vi "MCP4725 Example 1.vi"(8 "Error In":errorcluster) -> (0 "Error Out":errorcluster)   [LabVIEW 2014, in "LabVIEW Universal Transcriptor MCP4725.lvlib"]
uses:
  LabVIEW Universal Transcriptor MCP4725.lvlib
  MCP4725.lvclass
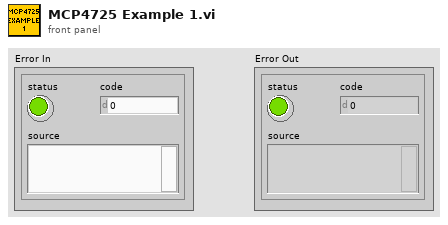
[diagram p1: front panel]
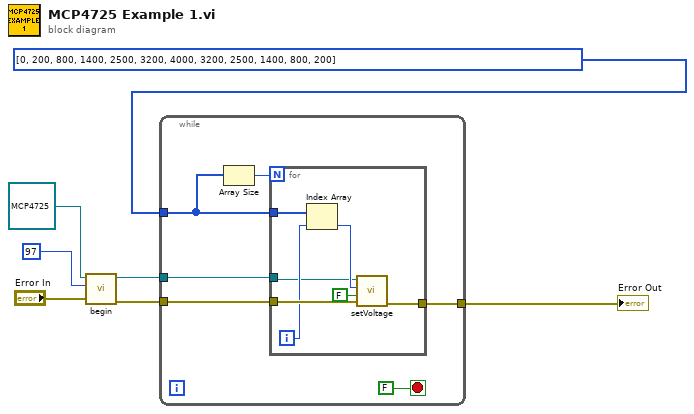
[diagram p0: block diagram]
diagram:
  n1 = call "begin.vi"("error in (no error)"="Error In", "I2C addr"=u8 97, "MCP4725 in"=refnum<class "MCP4725.lvclass"> refnum) -> ("error out"=w5:errorcluster, "MCP4725 out"=w4:refnum<class "MCP4725.lvclass">)  [unwired: 7 in]
  n2 = while {
    tunnel: w5 -> [w12]
    tunnel: w4 -> [w11]
    tunnel: u16[] [0, 200, 800, 1400, 2500, 3200, 4000, 3200, 2500, 1400, 800, 200] -> [w10]
    tunnel: [w8] -> w2
    stop <- FALSE stop-if-true
    n3 = Array Size(array=w10) -> (size(s)=w9:i32)
    n4 = for {
      N: w9 -> [_]
      tunnel: w12 -> [w20]
      tunnel: w11 -> [w16]
      tunnel: w10 -> [w19]
      tunnel: [w15] -> w8
      i -> [w18]
      n5 = Index Array(array=w19, index=w18) -> (element=w17:u16)
      n6 = call "setVoltage.vi"("error in (no error)"=w20, "writeEEPROM?"=FALSE, "voltage"=w17, "MCP4725 in"=w16) -> ("error out"=w15:errorcluster)  [unwired: 6 in, 1 out]
    }
  }
  "Error Out" <- w2
